vi "Population ReInit.vi"(8 "error in (no error)":errorcluster, 11 "TSP Class in":refnum<class "TSP Class.lvclass">) -> (0 "error out":errorcluster, 3 "TSP Class out":refnum<class "TSP Class.lvclass">)   [LabVIEW 2015, in "TSP Library.lvlib" / "TSP Class.lvclass"]
uses:
  TSP Class.lvclass
  TypeDef/Path.ctl
  TypeDef/Coordinate.ctl
  TSP Class.lvclass/TSP Class.ctl
  TSP Library.lvlib
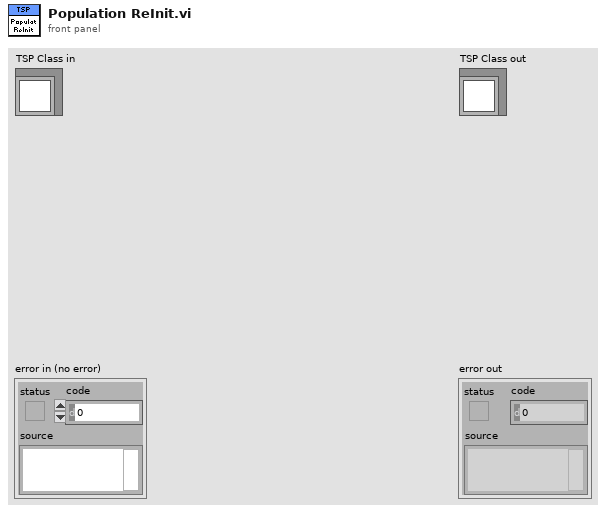
[diagram p1: front panel]
types:
  T1 = typedef "TSP Library.lvlib/Path.ctl" = cluster{"Distance":dbl, "Coordinate[]":T2[]}
  T2 = typedef "TSP Library.lvlib/Coordinate.ctl" = cluster{"x":dbl, "y":dbl}
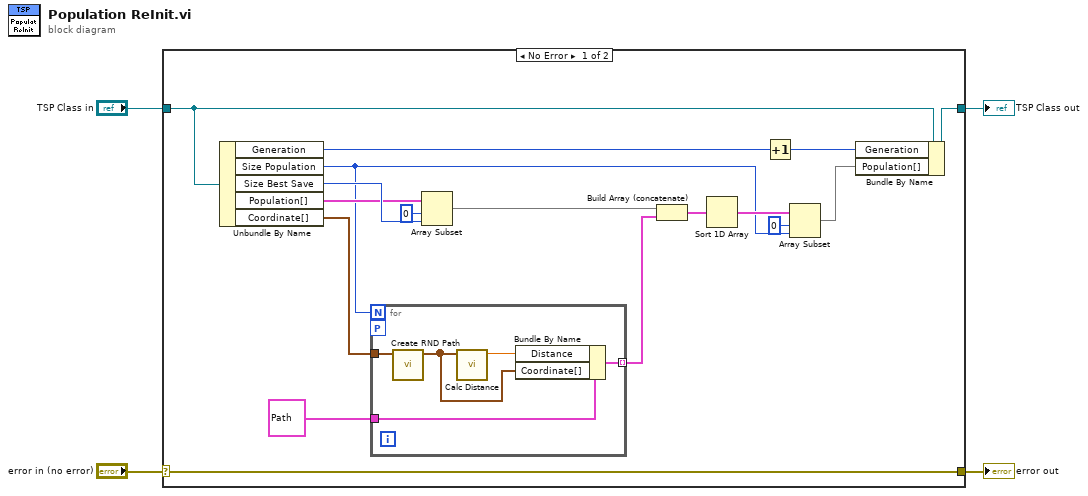
[diagram p0: block diagram]
diagram:
  n1 = case shown="No Error" "error in (no error)" {
    selector: "error in (no error)" -> [w21 w28]
    tunnel: [w21 w28] -> w3
    tunnel: [w19 w27] -> w1
    tunnel: "TSP Class in" -> [w10 w27]
    frame No Error {
      n2 = Unbundle By Name(w10) -> ("Generation"=w11:u64, "Size Population"=w6:u16, "Size Best Save"=w17:u16, "Population[]"=w16:T1[], "Coordinate[]"=w5:T2[])
      n3 = for {
        N: w6 -> [_]
        tunnel: w5 -> [w26]
        tunnel: T1 {"Distance"=0.0, "Coordinate[]"=[{"x"=67.57906304229073, "y"=68.60831518225434}, {"x"=81.83522625397705, "y"=7.983158550148239}, {"x"=13.845000200345314, "y"=50.20462870854803}, {"x"=65.60632392598347, "y"=23.41592963463568}, {"x"=37.527186631799125, "y"=49.26560940206024}, {"x"=75.80408834272797, "y"=82.83507884873025}, {"x"=91.24590880296392, "y"=43.00621931342281}, {"x"=88.66715419959786, "y"=61.38804665807669}, {"x"=86.51526432096372, "y"=8.714647141634234}, {"x"=83.91892871742184, "y"=30.341190073224354}, {"x"=24.743038312024, "y"=79.88068424696041}, {"x"=25.30168704115323, "y"=47.03932115592622}, {"x"=88.22800157317587, "y"=11.43101038338128}]} ("Path") -> [w25]
        tunnel: [w22] -> w7 mode=indexing
        workers-P: _ -> [_]
        n4 = call "Create RND Path.vi"("Coordinate[] In"=w26) -> ("Coordinate[] Out"=w23:T2[])  [unwired: 10 in]
        n5 = call "Calc Distance.vi"("Coordinate[] In"=w23) -> ("Distance"=w24:dbl)  [unwired: 10 in]
        n6 = Bundle By Name(cluster=w25, "Distance"=w24, "Coordinate[]"=w23) -> (w22:T1)
      }
      n7 = Array Subset(array=w16, index=0, length=w17) -> (w15:T1[])
      n8 = Build Array (concatenate)(w15, w7) -> (w14:T1[])
      n9 = Sort 1D Array(array=w14) -> (sorted array=w12:T1[])
      n10 = Increment(x=w11) -> (x+1=w9:u64)
      n11 = Array Subset(array=w12, index=0, length=w6) -> (w8:T1[])
      n12 = Bundle By Name(cluster=w10, "Generation"=w9, "Population[]"=w8) -> (w19:refnum<class "TSP Class.lvclass">)
    }
    frame Error {
    }
  }
  "error out" <- w3
  "TSP Class out" <- w1
